vi "Meas Add Temperature Data To Sample MAT File.vi"(8 "error in":errorcluster, 10 "aux data":T1, 11 "MAT file ref in":refnum<file>) -> (0 "error out":errorcluster, 3 "MAT file ref out":refnum<file>)   [LabVIEW 2018]
doc: "Write logged temperature data to the samples MAT file. It will write the data even if they are empty."
uses:
  adc/ADC Aux Data.ctl
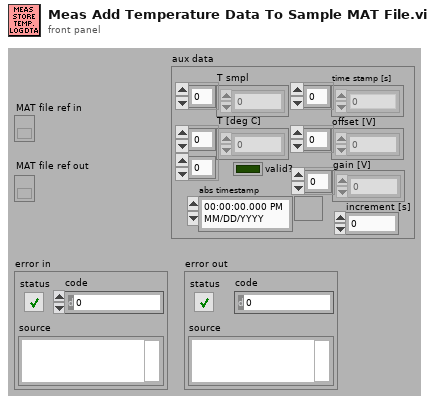
[diagram p1: front panel]
types:
  T1 = typedef "ADC Aux Data.ctl" = cluster{"offset [V]":dbl[], "gain [V]":dbl[], "time stamp [s]":dbl[], "increment [s]":dbl, "T smpl":i64[], "T [deg C]":dbl[][], "valid?":bool, "abs timestamp":timestamp}
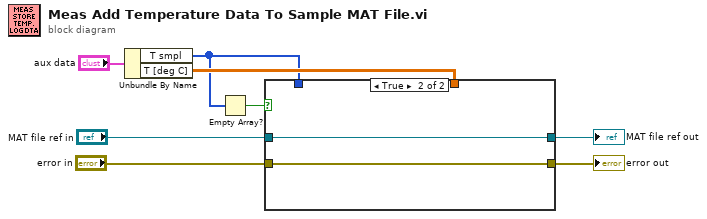
[diagram p0: block diagram]
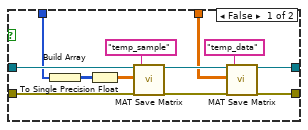
[diagram p2: hidden frame]
diagram:
  n1 = Unbundle By Name("aux data") -> ("T smpl"=w1:i64[], "T [deg C]"=w5:dbl[][])
  n2 = Empty Array?(array=w1) -> (empty?=w2:bool)
  n3 = case shown="True" w2 {
    tunnel: "error in" -> [w20 w22]
    tunnel: "MAT file ref in" -> [w19 w21]
    tunnel: w5 -> [w14 _]
    tunnel: w1 -> [w13 _]
    tunnel: [w10 w22] -> w4
    tunnel: [w9 w21] -> w3
    frame False {
      n4 = Build Array(w13) -> (w12:i64[][])
      n5 = To Single Precision Float(number=w12) -> (single precision float=w11:sgl[][])
      n6 = call "MAT Save Matrix.vi"("Ref Num"=w19, "SGL"=w11, "error in"=w20, "Matrix Name"="temp_sample") -> ("Dup Ref Num"=w15:refnum<file>, "error out"=w16:errorcluster)  [unwired: 14 in]
      n7 = call "MAT Save Matrix.vi"("Ref Num"=w15, "SGL"=w14, "error in"=w16, "Matrix Name"="temp_data") -> ("Dup Ref Num"=w9:refnum<file>, "error out"=w10:errorcluster)  [unwired: 14 in]
    }
    frame True {
    }
  }
  "error out" <- w4
  "MAT file ref out" <- w3
